vi "CheckFormClose.vi"(8 "エラー入力（エラーなし）":errorcluster, 10 "確認メッセージ表示?":bool, 11 "子画面Ref配列":refnum<vi>[](array[refnum])) -> (0 "エラー出力":errorcluster, 2 "終了可能":bool)   [LabVIEW 2014]
panel:
  # "子画面実行中なら、エラーとしてダイアログ表示する"
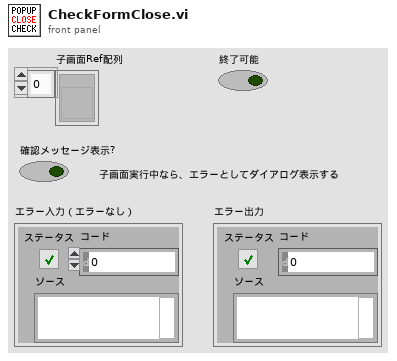
[diagram p1: front panel]
types:
  T1 = enum16{"PopUp", "GetParam", "SetParam", "RunCheck"}
  T2 = enum32{"Bad", "Idle", "Run top level", "Running"}
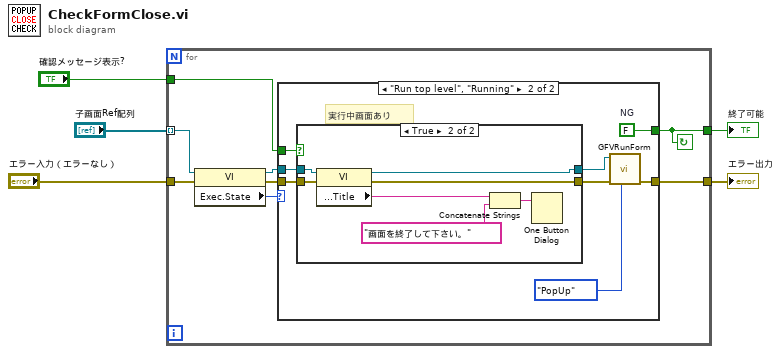
[diagram p0: block diagram]
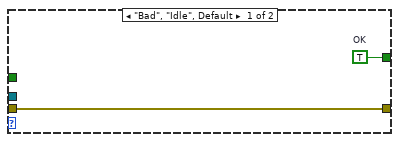
[diagram p2: hidden frame]
diagram:
  n1 = for {
    tunnel: "子画面Ref配列" -> [w13] mode=indexing
    tunnel: "エラー入力（エラーなし）" -> [w12]
    tunnel: [w10] -> w3
    tunnel: [w7] -> w4
    tunnel: "確認メッセージ表示?" -> [w6]
    stop <- w7 continue-if-true
    n2 = property class="VI"(reference=w13, error in=w12) -> (reference out=w8:refnum<vi>, error out=w9:errorcluster, "Exec.State"=w11:T2)
    n3 = case shown="\"Run top level\", \"Running\"" w11 {
      tunnel: [w15 w18] -> w10
      tunnel: w9 -> [w15 w22]
      tunnel: w8 -> [_ w23]
      tunnel: [w14 w21] -> w7
      tunnel: w6 -> [_ w16]
      frame "Bad", "Idle", Default {
        w14 = TRUE  # OK
      }
      frame "Run top level", "Running" {
        w21 = FALSE  # NG
        # "実行中画面あり"
        n4 = case shown="TRUE" w16 {
          tunnel: w23 -> [w25 w32]
          tunnel: w22 -> [w24 w31]
          tunnel: [w24 w27] -> w20
          tunnel: [w25 w26] -> w19
          frame False {
          }
          frame True {
            n5 = property class="VI"(reference=w32, error in=w31) -> (reference out=w26:refnum<vi>, error out=w27:errorcluster, "Front Panel.Title"=w30:string)
            n6 = Concatenate Strings(w30, "画面を終了して下さい。") -> (w28:string)
            n7 = One Button Dialog(message=w28) -> ()  [unwired: 1 in, 1 out]
          }
        }
        n8 = call "GFVRunForm.vi"("Mode"=T1."PopUp", "エラー入力(エラーなし)"=w20, "VI refnum"=w19) -> ("エラー出力"=w18:errorcluster)  [unwired: 3 in, 5 out]
      }
    }
  }
  "終了可能" <- w4
  "エラー出力" <- w3
